vi "FdxCmdTxQueueWriteCvi.vi"(8 "error in":errorcluster, 9 "TxQueueWriteIn":T1 {"FrameType" items=["FDX_TX_FRAME_STD", "FDX_TX_FRAME_INSTR"]; "SequenceNumberOffset" items=["FDX_TX_FRAME_SEQ_OFFS_AUTO "=65535]; "SequenceNumberInit" items=["FDX_TX_FRAME_SEQ_INIT_AUTO"=65535]; "PhysErrorInjection" items=["FDX_TX_FRAME_ERR_OFF"=0, "FDX_TX_FRAME_ERR_CRC"=1, "FDX_TX_FRAME_ERR_ALI"=2, "FDX_TX_FRAME_ERR_PRE"=4, "FDX_TX_FRAME_ERR_PHY"=8]; "FrameStartMode" items=["FDX_TX_FRAME_START_IFG", "FDX_TX_FRAME_START_PGWT", "FDX_TX_FRAME_START_TRG"]; "NetSelect" items=["FDX_TX_FRAME_DLY_A"=0, "FDX_TX_FRAME_DLY_B"=1, "FDX_TX_FRAME_BOTH "=3, "FDX_TX_FRAME_ONLY_A"=4, "FDX_TX_FRAME_ONLY_B "=5]; "PreambleCount" max=15; "ExternalStrobe" items=["FDX_DIS", "FDX_ENA"]; "PayloadGenerationMode" items=["FDX_TX_FRAME_PGM_USER"=0, "FDX_TX_FRAME_PGM_IP_PART"=1, "FDX_TX_FRAME_PGM_IP_FULL"=2, "FDX_TX_FRAME_PGM_IP_PART_TT"=10, "FDX_TX_FRAME_PGM_IP_FULL_TT"=20]; "PayloadBufferMode" items=["FDX_TX_FRAME_PBM_STD", "FDX_TX_FRAME_PBM_MAC", "FDX_TX_FRAME_PBM_UDP"]; "HeaderType" items=["FDX_TX_FRAME_HEADER_GENERIC ", "FDX_TX_FRAME_HEADER_REPLAY"]}, 11 "InstrumentHandle_port":u32) -> (0 "error out":errorcluster, 3 "InstrumentHandle_port":u32)   [LabVIEW 2020, in "AIM664LV.lvlib"]
doc: "This function is used to write Entries to a Transmit Queue from a provided buffer. For this write function the number of Entries and the number of bytes to write needs to be specified. The entries will always be queued at the end of the transmit queue."
uses:
  AIM664LV.lvlib
  AFDX_LibraryAdmin/FdxGlobalDllPath.vi
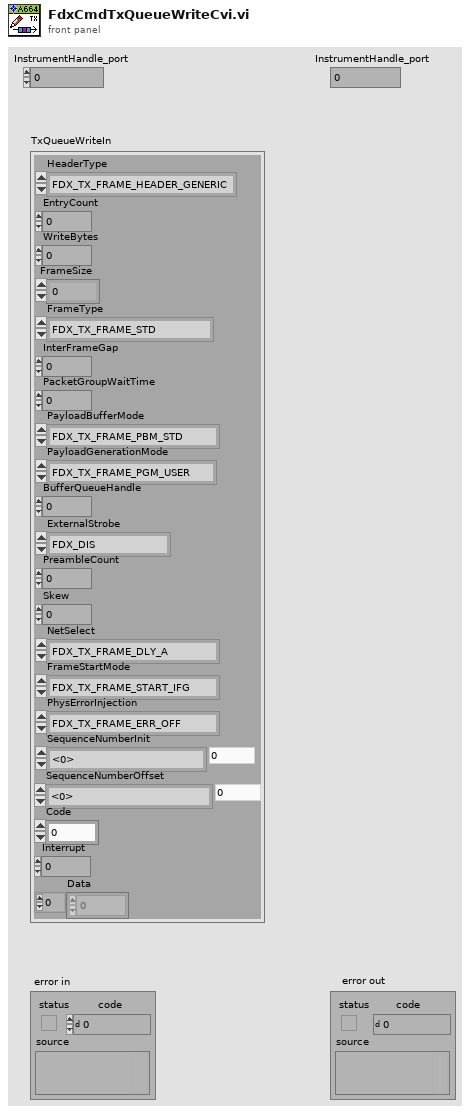
[diagram p1: front panel]
types:
  T1 = cluster{"HeaderType":u32, "EntryCount":u32, "WriteBytes":u32, "FrameSize":u16, "FrameType":u8, "InterFrameGap":u32, "PacketGroupWaitTime":u32, "PayloadBufferMode":u8, "PayloadGenerationMode":u8, "BufferQueueHandle":u32, "ExternalStrobe":u8, "PreambleCount":u8, "Skew":u32, "NetSelect":u8, "FrameStartMode":u8, "PhysErrorInjection":u32, "SequenceNumberInit":u16, "SequenceNumberOffset":u16, "Code":u8, "Interrupt":u8, "Data":u8[]}
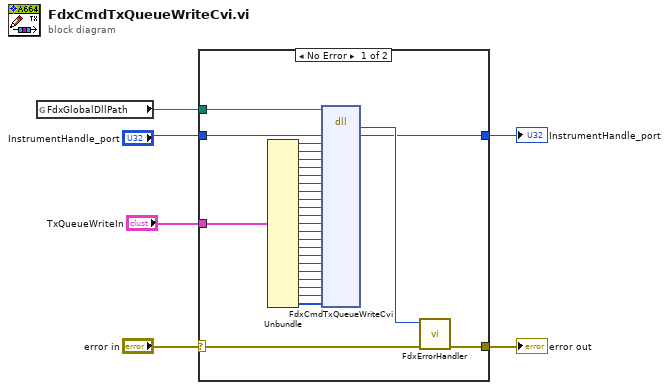
[diagram p0: block diagram]
diagram:
  n1 = global read "FdxGlobalDllPath.vi" "FdxGlobalDllPath"() -> (w4:path)
  n2 = case shown="No Error" "error in" {
    selector: "error in" -> [w33 w36]
    tunnel: [w34 w36] -> w6
    tunnel: w4 -> [w10 _]
    tunnel: [w9 w35] -> w3
    tunnel: "InstrumentHandle_port" -> [w8 w35]
    tunnel: "TxQueueWriteIn" -> [w7 _]
    frame No Error {
      n3 = Unbundle(w7) -> ("HeaderType"=w31:u32, "EntryCount"=w30:u32, "WriteBytes"=w29:u32, "FrameSize"=w28:u16, "FrameType"=w27:u8, "InterFrameGap"=w26:u32, "PacketGroupWaitTime"=w25:u32, "PayloadBufferMode"=w24:u8, "PayloadGenerationMode"=w23:u8, "BufferQueueHandle"=w22:u32, "ExternalStrobe"=w21:u8, "PreambleCount"=w20:u8, "Skew"=w19:u32, "NetSelect"=w18:u8, "FrameStartMode"=w17:u8, "PhysErrorInjection"=w16:u32, "SequenceNumberInit"=w15:u16, "SequenceNumberOffset"=w14:u16, "Code"=w13:u8, "Interrupt"=w12:u8, "Data"=w11:u8[])
      n4 = dll-call lib="aim_fdx.19.dll" fn="FdxCmdTxQueueWriteCvi"(path in=w10, "InstrumentHandle"=w8, "HeaderType"=w31, "EntryCount"=w30, "WriteBytes"=w29, "uw_FrameSize"=w28, "uc_FrameType"=w27, "ul_InterFrameGap"=w26, "ul_PacketGroupWaitTime"=w25, "uc_PayloadBufferMode"=w24, "uc_PayloadGenerationMode"=w23, "ul_BufferQueueHandle"=w22, "uc_ExternalStrobe"=w21, "uc_PreambleCount"=w20, "ul_Skew"=w19, "uc_NetSelect"=w18, "uc_FrameStartMode"=w17, "ul_PhysErrorInjection"=w16, "uw_SequenceNumberInit"=w15, "uw_SequenceNumberOffset"=w14, "uc_Code"=w13, "uc_Interrupt"=w12, "Data"=w11) -> ("status"=w32:i32, "InstrumentHandle"=w9:u32)  [unwired: 23 in, 2 out]
      n5 = call "FdxErrorHandler.vi"("error in"=w33, "AIM Error"=w32) -> ("error out"=w34:errorcluster)  [unwired: 9 in]
    }
    frame Error {
    }
  }
  "error out" <- w6
  "InstrumentHandle_port" <- w3
